vi "Dpc Set Tms Tdi Tck.vi"(0 "hif":u32, 1 "perc":i32, 5 "fTms":i32, 7 "fTdi":i32, 9 "fTck":i32, 11 "error in (no error)":errorcluster, 12 "ptrid":u16) -> (3 "perc out":i32, 4 "hif out":u32, 6 "function return":i32, 14 "ptrid out":u16, 15 "error out":errorcluster)   [LabVIEW 2011, in "LVH-Adept.lvlib" / "DPCUTIL.lvlib"]
doc: "DPCAPI BOOL DpcSetTmsTdiTck(HANDLE hif, BOOL fTms, BOOL fTdi, BOOL fTck, ERC * perc, TRID * ptrid);"
uses:
  DPCUTIL.lvlib
  dpcutil.dll
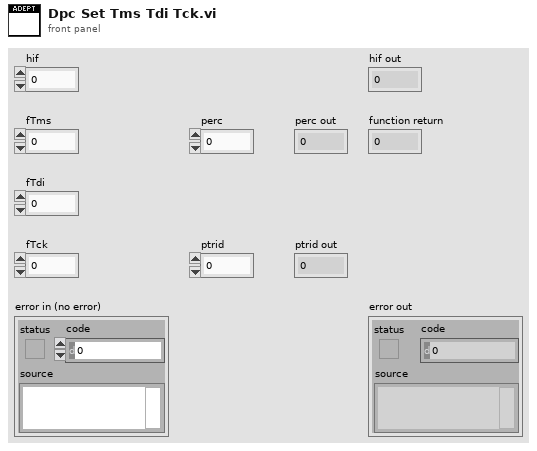
[diagram p1: front panel]
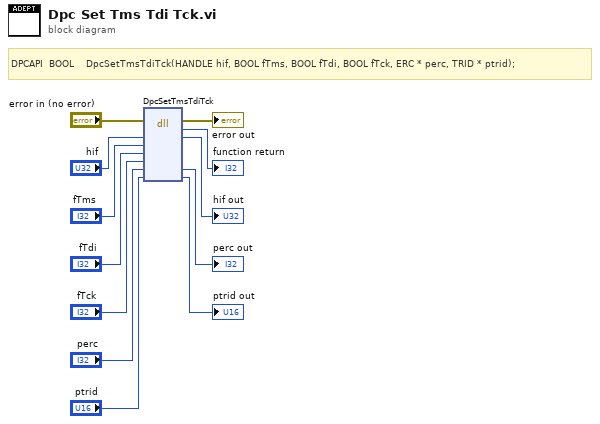
[diagram p0: block diagram]
diagram:
  # "DPCAPI  BOOL    DpcSetTmsTdiTck(HANDLE hif, BOOL fTms, BOOL fTdi, BOOL fTck, ERC * perc, TRID * ptrid);"
  n1 = dll-call lib="dpcutil.*" fn="DpcSetTmsTdiTck"(error in="error in (no error)", "hif"="hif", "fTms"="fTms", "fTdi"="fTdi", "fTck"="fTck", "perc"="perc", "ptrid"="ptrid") -> (error out=→"error out":errorcluster, →"function return":i32, "hif"=→"hif out":u32, "perc"=→"perc out":i32, "ptrid"=→"ptrid out":u16)  [unwired: 5 in, 1 out]
